vi "Get LVItem by Tag.vi"(8 "error in":errorcluster, 10 "Tag":string, 11 "Project in":refnum<class "Project.lvclass">) -> (0 "error out":errorcluster, 2 "Selected Library":refnum<class "Library.lvclass">, 3 "Selected VI":refnum<class "VI.lvclass">)   [LabVIEW 2019, in "Panther Dashboard.lvlib" / "Project.lvclass"]
uses:
  Project.lvclass
  Project.lvclass/Project.ctl
  LabVIEWItem/LabVIEWItem.lvclass/LabVIEWItem.ctl
  Library/Library.lvclass/Library.ctl
  LabVIEWItem/Read Item Tag.vi
  Read Libraries.vi
  Library/Read VIs MAP.vi
  Library/Library.lvclass
  VI/VI.lvclass
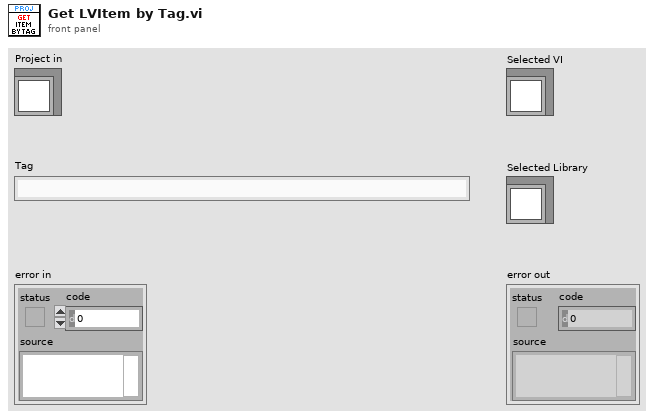
[diagram p1: front panel]
types:
  T1 = typedef "Panther Dashboard.lvlib/LabVIEWItem.lvclass/VI Type--enum.ctl" = enum16{"Requests", "Broadcasts", "Request and Wait for Reply", "Round Trip", "Public API VIs", "» Constant VIs", "» Error VIs", "Module", "Project"}
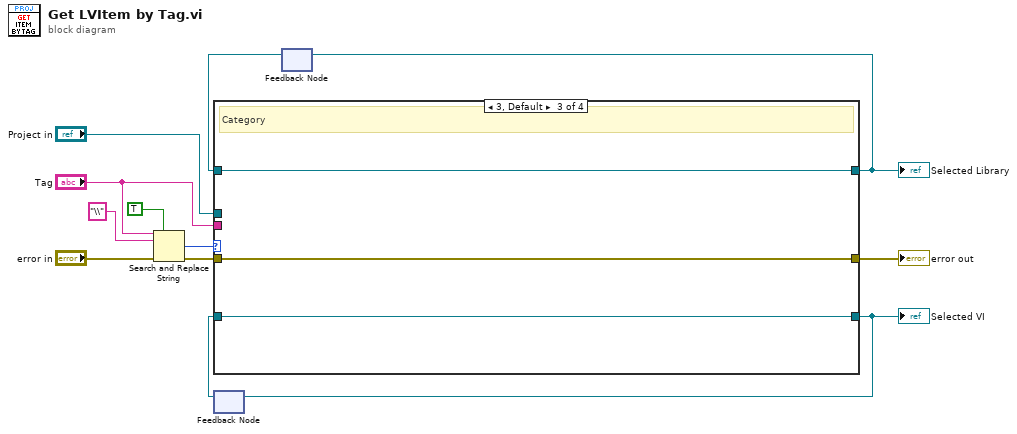
[diagram p0: block diagram]
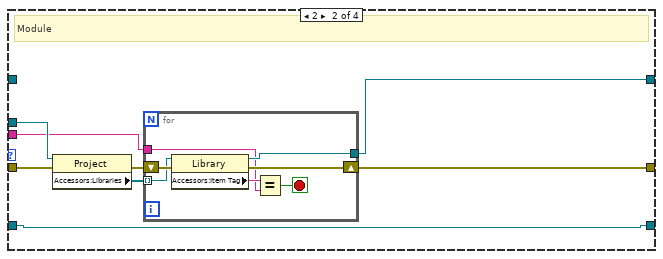
[diagram p3: hidden frame]
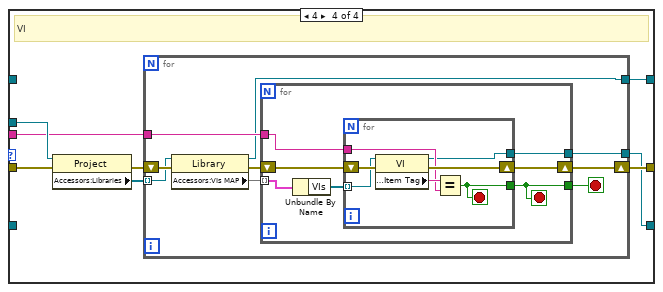
[diagram p4: hidden frame]
diagram:
  n1 = Search and Replace String(replace all?=TRUE ("replace all? (F)"), input string="Tag", search string="\\" ("Tag"), error in="error in") -> (number of replacements=w8:i32, error out=w11:errorcluster)  [unwired: 4 in, 2 out]
  n2 = feedback #1() -> (w1:refnum<class "VI.lvclass">)  [unwired: 1 in]
  n3 = feedback #2() -> (w3:refnum<class "Library.lvclass">)  [unwired: 1 in]
  n4 = case shown="3, Default" w8 {
    tunnel: w11 -> [w15 w23 w33 w41]
    tunnel: [w15 w21 w33 w39] -> w10
    tunnel: "Tag" -> [_ w18 _ w36]
    tunnel: "Project in" -> [_ w20 _ w38]
    tunnel: [w14 w17 w32 w35] -> w4
    tunnel: w3 -> [w14 _ w32 _]
    tunnel: [w13 w16 w31 w34] -> w2
    tunnel: w1 -> [w13 w16 w31 _]
    frame 1 {
      # "Project"
    }
    frame 2 {
      # "Module"
      n5 = property class="Project"(reference=w20, error in=w23) -> (error out=w22:errorcluster, "Accessors:Libraries"=w19:refnum<class "Library.lvclass">[])  [unwired: 1 out]
      n6 = for {
        tunnel: w19 -> [w28] mode=indexing
        tunnel: [w27] -> w17
        tunnel: w18 -> [w25]
        shift-right: [w29] -> w21
        shift-left: w22 -> [w30]
        stop <- w24 stop-if-true
        n7 = property class="Library"(reference=w28, error in=w30) -> (reference out=w27:refnum<class "Library.lvclass">, error out=w29:errorcluster, "Accessors:Item Tag"=w26:string)
        n8 = Equal?(x=w26, y=w25) -> (x = y?=w24:bool)
      }
    }
    frame 3, Default {
      # "Category"
    }
    frame 4 {
      # "VI"
      n9 = property class="Project"(reference=w38, error in=w41) -> (error out=w40:errorcluster, "Accessors:Libraries"=w37:refnum<class "Library.lvclass">[])  [unwired: 1 out]
      n10 = for {
        tunnel: w37 -> [w47] mode=indexing
        shift-right: [w48] -> w39
        shift-left: w40 -> [w50]
        tunnel: w36 -> [w45]
        tunnel: [w44] -> w34
        tunnel: [w42] -> w35
        stop <- w43 stop-if-true
        n11 = property class="Library"(reference=w47, error in=w50) -> (reference out=w42:refnum<class "Library.lvclass">, error out=w49:errorcluster, "Accessors:VIs MAP"=w46:map{T1, refnum<class "VI.lvclass">[]})
        n12 = for {
          tunnel: w46 -> [w55] mode=indexing
          shift-right: [w56] -> w48
          shift-left: w49 -> [w57]
          tunnel: w45 -> [w53]
          tunnel: [w52] -> w44
          tunnel: [w51] -> w43
          stop <- w51 stop-if-true
          n13 = Unbundle By Name(w55) -> ("VIs"=w54:refnum<class "VI.lvclass">[])
          n14 = for {
            tunnel: w54 -> [w62] mode=indexing
            shift-right: [w63] -> w56
            shift-left: w57 -> [w64]
            tunnel: w53 -> [w60]
            tunnel: [w59] -> w52
            tunnel: [w58] -> w51
            stop <- w58 stop-if-true
            n15 = property class="VI"(reference=w62, error in=w64) -> (reference out=w59:refnum<class "VI.lvclass">, error out=w63:errorcluster, "Accessors:Item Tag"=w61:string)
            n16 = Equal?(x=w61, y=w60) -> (x = y?=w58:bool)
          }
        }
      }
    }
  }
  "error out" <- w10
  "Selected VI" <- w2
  "Selected Library" <- w4
  n17 = feedback-in #1(w2) -> ()
  n18 = feedback-in #2(w4) -> ()
